vi "Memory Cell to float.vi"(7 "Field Selector":T1, 10 "Memory Cell":T2={"type"=enum."float", "x"=0.0, "y"=0.0, "z"=0.0, "w"=0.0}) -> (2 "float out":dbl)   [LabVIEW 2023]
uses:
  Type Definitions/Memory Cell.ctl
  Type Definitions/Memory Cell Type Enum.ctl
  Type Definitions/Cell Selector.ctl
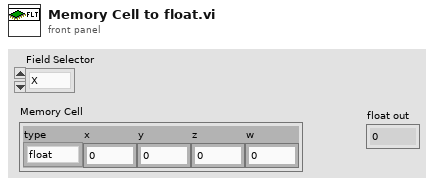
[diagram p1: front panel]
types:
  T1 = typedef "Cell Selector.ctl" = enum16{"X", "Y", "Z", "W"}
  T2 = typedef "Memory Cell.ctl" = cluster{"type":T3, "x":dbl, "y":dbl, "z":dbl, "w":dbl}
  T3 = typedef "Memory Cell Type Enum.ctl" = enum16{"integer", "float", "vector", "rotation"}
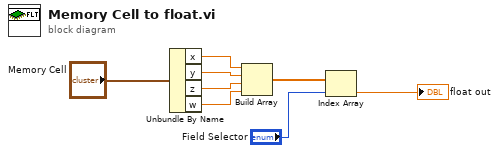
[diagram p0: block diagram]
diagram:
  n1 = Unbundle By Name("Memory Cell") -> ("x"=w7:dbl, "y"=w6:dbl, "z"=w5:dbl, "w"=w4:dbl)
  n2 = Build Array(w7, w6, w5, w4) -> (w3:dbl[])
  n3 = Index Array(array=w3, index="Field Selector") -> (element=→"float out":dbl)
